vi "verify_working_dir.vi"(8 "error in (no error)":errorcluster, 11 "working directory":path) -> (0 "error out":errorcluster, 3 "working directory out":path)   [LabVIEW 2013, in "dotnet_system_exec.lvclass"]
uses:
  dotnet_system_exec.lvclass
  <vilib>/Utility/sysdir.llb/System Directory Type.ctl
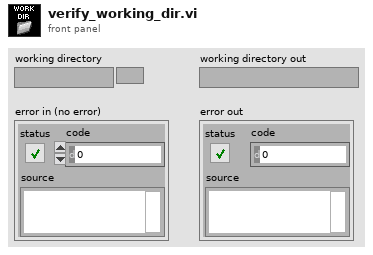
[diagram p1: front panel]
types:
  T1 = typedef "System Directory Type.ctl" = i32
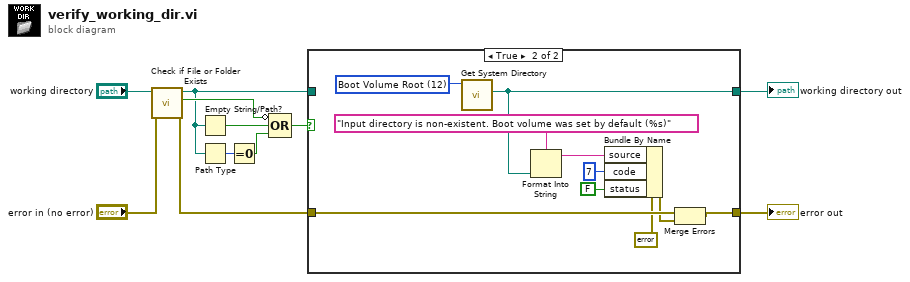
[diagram p0: block diagram]
diagram:
  n1 = call <vilib>:"Check if File or Folder Exists.vi"("error in (no error)"="error in (no error)", "path"="working directory") -> ("error out"=w7:errorcluster, "file or folder exists?"=w5:bool, "dup path"=w3:path)  [unwired: 7 in]
  n2 = Empty String/Path?(string/path=w3) -> (empty?=w4:bool)
  n3 = Path Type(1:w3) -> (0:w2:i16)
  n4 = Equal To 0?(x=w2) -> (x = 0?=w1:bool)
  n5 = Compound Arithmetic op=OR(invert w5, w4, w1) -> (w6:bool)
  n6 = case shown="True" w6 {
    tunnel: w3 -> [w12 _]
    tunnel: [w12 w21] -> w10
    tunnel: w7 -> [w13 w22]
    tunnel: [w13 w23] -> w11
    frame False {
    }
    frame True {
      w16 = T1 12 items=["User Home"=0, "User Desktop"=1, "User Documents"=2, "User Application Data"=3, "User Preferences"=4, "User Temporary"=5, "Public Documents"=6, "Public Application Data"=7, "Public Preferences"=8, "Public Cache"=13, "System Core Libraries"=9, "System Installed Libraries"=10, "Application Files"=11, "Boot Volume Root"=12] ("system directory type")
      n7 = call <vilib>:"Get System Directory.vi"("system directory type"=w16) -> ("system directory"=w21:path)  [unwired: 10 in]
      n8 = Format Into String(format string="Input directory is non-existent. Boot volume was set by default (%s)", w21) -> (resulting string=w15:string)  [unwired: 2 in, 1 out]
      n9 = Bundle By Name(cluster=errorcluster {"status"=FALSE, "code"=0, "source"=""} ("error in"), "source"=w15, "code"=7, "status"=FALSE) -> (w19:errorcluster)
      n10 = Merge Errors(w22, w19) -> (w23:errorcluster)
    }
  }
  "error out" <- w11
  "working directory out" <- w10
